vi "FGV_DOCK_multistate_indicator.vi"(6 "boolean_indicator_refnum":refnum<vi>, 7 "options":T1, 8 "error_in":errorcluster) -> (0 "error_out":errorcluster)   [LabVIEW 2019]
uses:
  FGV_DOCK_multistate_indicator.ctl
  state_triggers.ctl
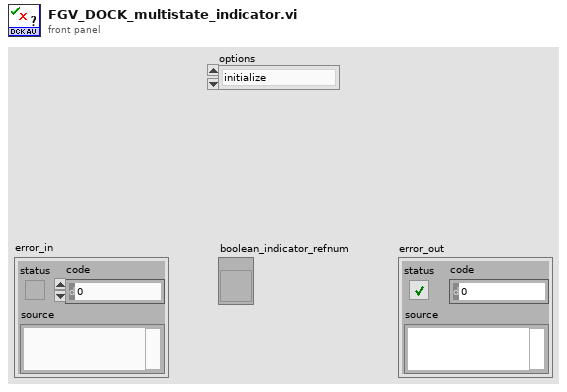
[diagram p1: front panel]
types:
  T1 = typedef "FGV_DOCK_multistate_indicator.ctl" = enum16{"initialize", "login", "logout", "start_batch", "finish_batch", "gear_OK", "gear_NOK", "gear_clear", "translate", "error", "error_clear"}
  T2 = typedef "state_triggers.ctl" = cluster{"logged_in?":bool, "batch_active?":bool, "error_active?":bool, "gear_loaded?":bool, "gear_ok?":bool}
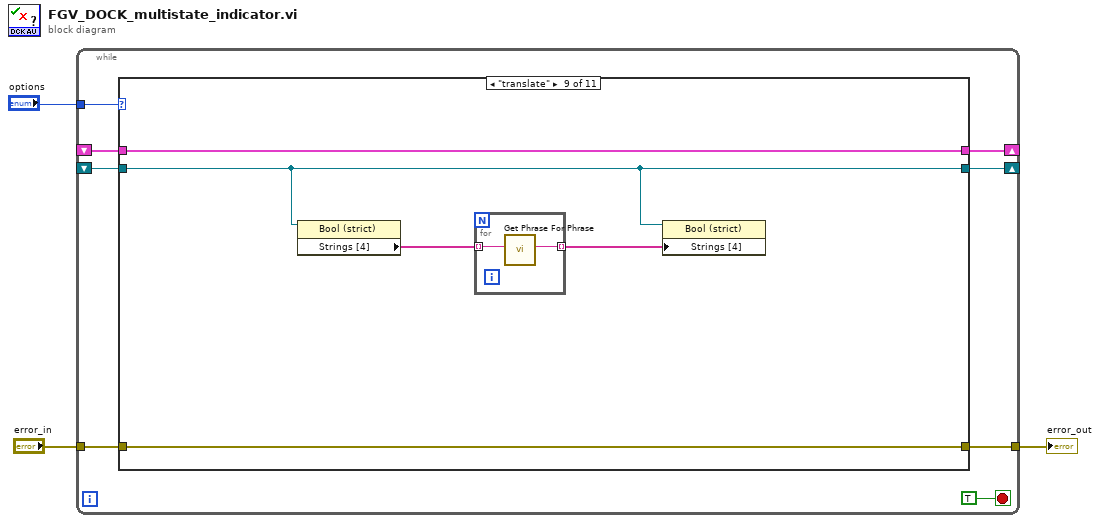
[diagram p0: block diagram]
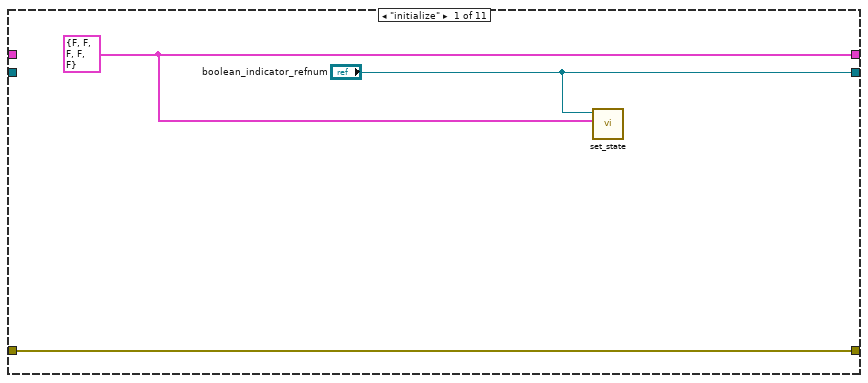
[diagram p2: hidden frame]
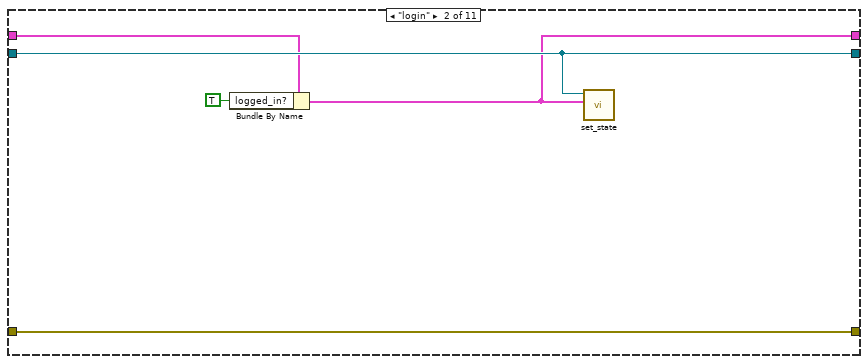
[diagram p3: hidden frame]
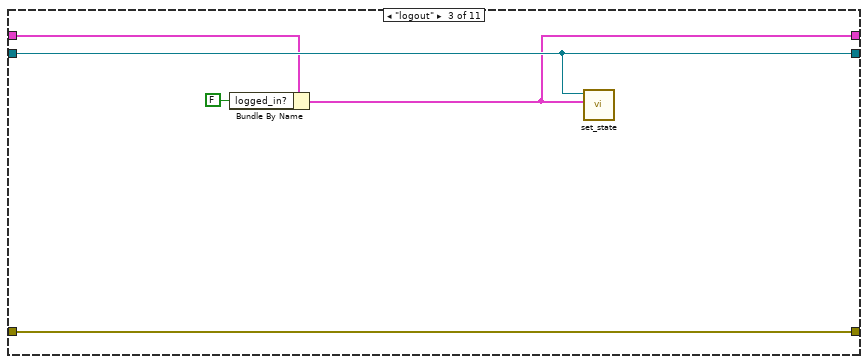
[diagram p4: hidden frame]
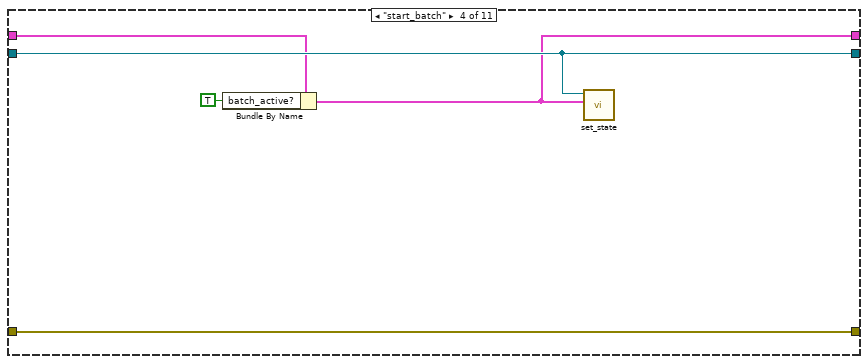
[diagram p5: hidden frame]
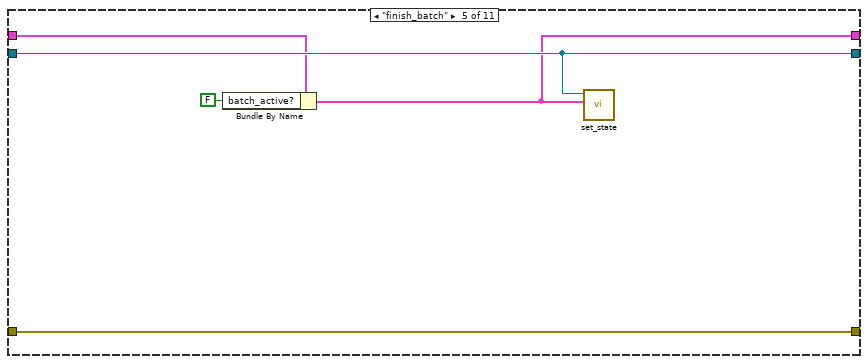
[diagram p6: hidden frame]
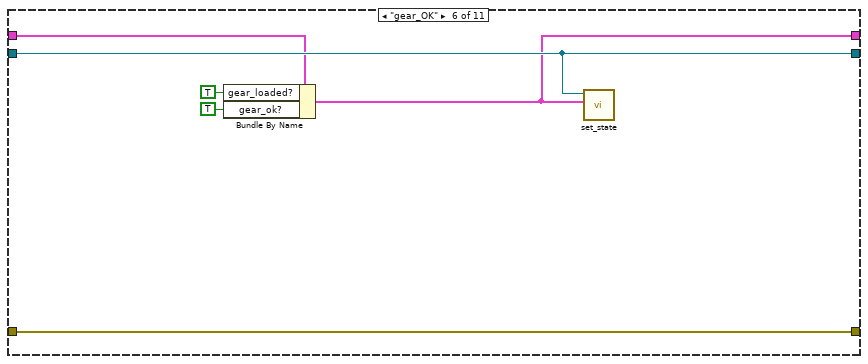
[diagram p7: hidden frame]
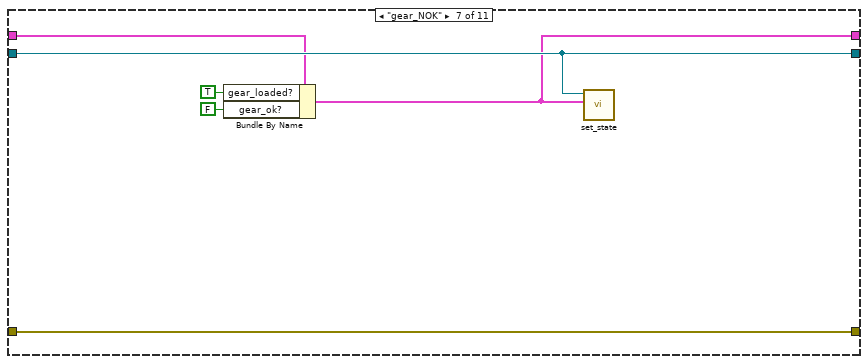
[diagram p8: hidden frame]
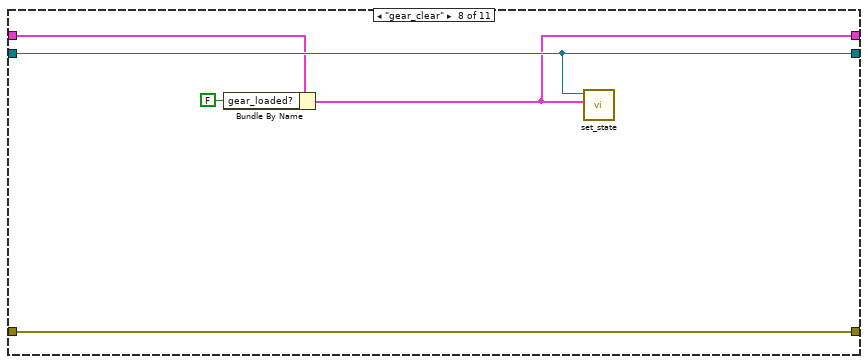
[diagram p9: hidden frame]
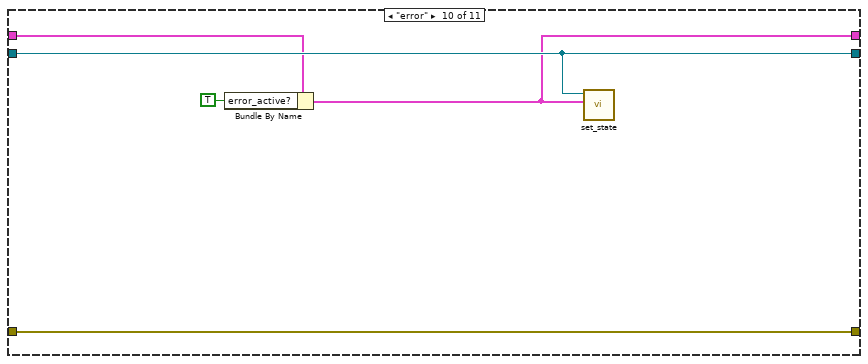
[diagram p10: hidden frame]
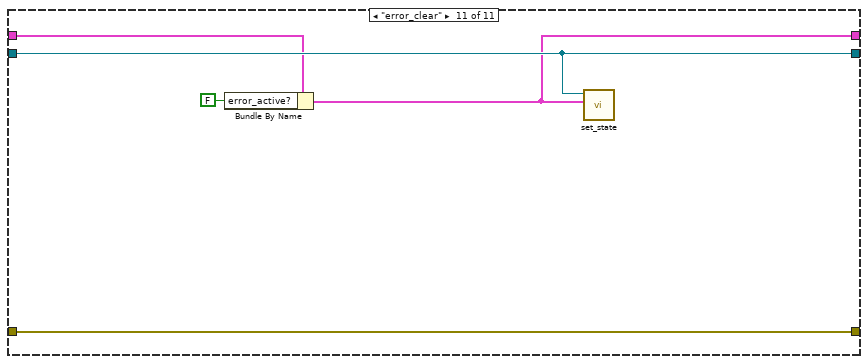
[diagram p11: hidden frame]
diagram:
  n1 = while {
    tunnel: "options" -> [w10]
    tunnel: [w9] -> w3
    tunnel: "error_in" -> [w8]
    shift-right: [w7] -> _
    shift-left: _ -> [w6]
    shift-right: [w5] -> _
    shift-left: _ -> [w4]
    stop <- TRUE stop-if-true
    n2 = case shown="\"translate\"" w10 {
      tunnel: [w14 w19 w24 w29 w34 w40 w46 w51 w52 w63 w68] -> w9
      tunnel: w8 -> [w14 w19 w24 w29 w34 w40 w46 w51 w52 w63 w68]
      tunnel: ["boolean_indicator_refnum" w18 w23 w28 w33 w39 w45 w50 w53 w62 w67] -> w7
      tunnel: w6 -> [_ w18 w23 w28 w33 w39 w45 w50 w53 w62 w67]
      tunnel: [w12 w15 w20 w25 w30 w36 w42 w47 w56 w59 w64] -> w5
      tunnel: w4 -> [_ w17 w22 w27 w32 w38 w44 w49 w56 w61 w66]
      frame "initialize" {
        w12 = T2 {"logged_in?"=FALSE, "batch_active?"=FALSE, "error_active?"=FALSE, "gear_loaded?"=FALSE, "gear_ok?"=FALSE} ("state_triggers")
        n3 = call "set_state.vi"("boolean_indicator_refnum"="boolean_indicator_refnum", "state_triggers"=w12) -> ()  [unwired: 9 in]
      }
      frame "login" {
        n4 = Bundle By Name(cluster=w17, "logged_in?"=TRUE) -> (w15:T2)
        n5 = call "set_state.vi"("boolean_indicator_refnum"=w18, "state_triggers"=w15) -> ()  [unwired: 9 in]
      }
      frame "logout" {
        n6 = Bundle By Name(cluster=w22, "logged_in?"=FALSE) -> (w20:T2)
        n7 = call "set_state.vi"("boolean_indicator_refnum"=w23, "state_triggers"=w20) -> ()  [unwired: 9 in]
      }
      frame "start_batch" {
        n8 = Bundle By Name(cluster=w27, "batch_active?"=TRUE ("logged_in?")) -> (w25:T2)
        n9 = call "set_state.vi"("boolean_indicator_refnum"=w28, "state_triggers"=w25) -> ()  [unwired: 9 in]
      }
      frame "finish_batch" {
        n10 = Bundle By Name(cluster=w32, "batch_active?"=FALSE ("logged_in?")) -> (w30:T2)
        n11 = call "set_state.vi"("boolean_indicator_refnum"=w33, "state_triggers"=w30) -> ()  [unwired: 9 in]
      }
      frame "gear_OK" {
        n12 = Bundle By Name(cluster=w38, "gear_loaded?"=TRUE ("logged_in?"), "gear_ok?"=TRUE) -> (w36:T2)
        n13 = call "set_state.vi"("boolean_indicator_refnum"=w39, "state_triggers"=w36) -> ()  [unwired: 9 in]
      }
      frame "gear_NOK" {
        n14 = Bundle By Name(cluster=w44, "gear_loaded?"=TRUE ("logged_in?"), "gear_ok?"=FALSE) -> (w42:T2)
        n15 = call "set_state.vi"("boolean_indicator_refnum"=w45, "state_triggers"=w42) -> ()  [unwired: 9 in]
      }
      frame "gear_clear" {
        n16 = Bundle By Name(cluster=w49, "gear_loaded?"=FALSE ("logged_in?")) -> (w47:T2)
        n17 = call "set_state.vi"("boolean_indicator_refnum"=w50, "state_triggers"=w47) -> ()  [unwired: 9 in]
      }
      frame "translate" {
        n18 = property on="Property Node" class="Bool (strict)"(reference=w53) -> ("Strings [4]"=w55:string[])  [unwired: 1 in, 2 out]
        n19 = for {
          tunnel: w55 -> [w58] mode=indexing
          tunnel: [w57] -> w54 mode=indexing
          n20 = call "Get Phrase For Phrase.vi"("Phrase"=w58) -> ("Phrase"=w57:string)  [unwired: 9 in, 1 out]
        }
        n21 = property on="Property Node" class="Bool (strict)"(reference=w53, "Strings [4]"=w54) -> ()  [unwired: 1 in, 2 out]
      }
      frame "error" {
        n22 = Bundle By Name(cluster=w61, "error_active?"=TRUE ("logged_in?")) -> (w59:T2)
        n23 = call "set_state.vi"("boolean_indicator_refnum"=w62, "state_triggers"=w59) -> ()  [unwired: 9 in]
      }
      frame "error_clear" {
        n24 = Bundle By Name(cluster=w66, "error_active?"=FALSE ("logged_in?")) -> (w64:T2)
        n25 = call "set_state.vi"("boolean_indicator_refnum"=w67, "state_triggers"=w64) -> ()  [unwired: 9 in]
      }
    }
  }
  "error_out" <- w3
